vi "approximate fraction (powers of 2).vi"() -> ()   [LabVIEW 2009]
panel:
  out "whole":i32
  out "numerator":dbl format="%.2f"
  in  "Decimal":dbl
  in  "Accuracy":u8(ring) items=["1/2", "1/4", "1/8", "1/16", "1/32", "1/64", "1/128"]
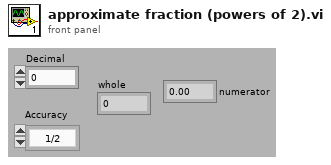
[diagram p1: front panel]
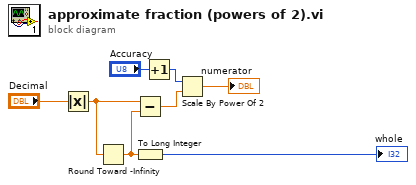
[diagram p0: block diagram]
diagram:
  n1 = Absolute Value(x="Decimal") -> (abs(x)=w6:dbl)
  n2 = Round Toward -Infinity(1:w6) -> (0:w7:dbl)
  n3 = Subtract(x=w6, y=w7) -> (x-y=w2:dbl)
  n4 = To Long Integer(number=w7) -> (32bit integer=→"whole":i32)
  n5 = Increment(x="Accuracy") -> (x+1=w3:u8)
  n6 = Scale By Power Of 2(n=w3, x=w2) -> (x*2^n=→"numerator":dbl)
